vi "4461 - Lockin Engine.vi"(8 "error in (no error)":errorcluster, 9 "Reference In":waveform(dbl)[](array[waveform]), 10 "Signal in":waveform(dbl)[](array[waveform]), 11 "Lockin":refnum<class "Instrument.Lockin.lvclass">) -> (0 "error out":errorcluster, 1 "filter fC (Hz)":dbl=0.3183098861837907, 2 "Results (X,Y,R,Theta)":dbl[][](array[numeric]), 3 "Lockin out":refnum<class "Instrument.Lockin.lvclass">)   [LabVIEW 2016, in "LockinDAQ.lvclass"]
uses:
  LockinDAQ.lvclass
  <vilib>/Analysis/NI_AALBase.lvlib
  <vilib>/Analysis/baseanly.llb/Mean (DBL).vi
  Instrument.Lockin/Instrument.Lockin.lvclass
  C:/Program Files (x86)/National Instruments/LabVIEW 2016/user.lib/LevyLab/Levylab Instruments/SMOs/Instrument/Instrument.lvclass
  C:/Program Files (x86)/National Instruments/LabVIEW 2016/user.lib/LevyLab/Levylab Instruments/SMOs/LevyLab/LevyLab.lvclass
  C:/Program Files (x86)/National Instruments/LabVIEW 2016/vi.lib/JKI/JKI SMO/SMO/SMO.lvclass
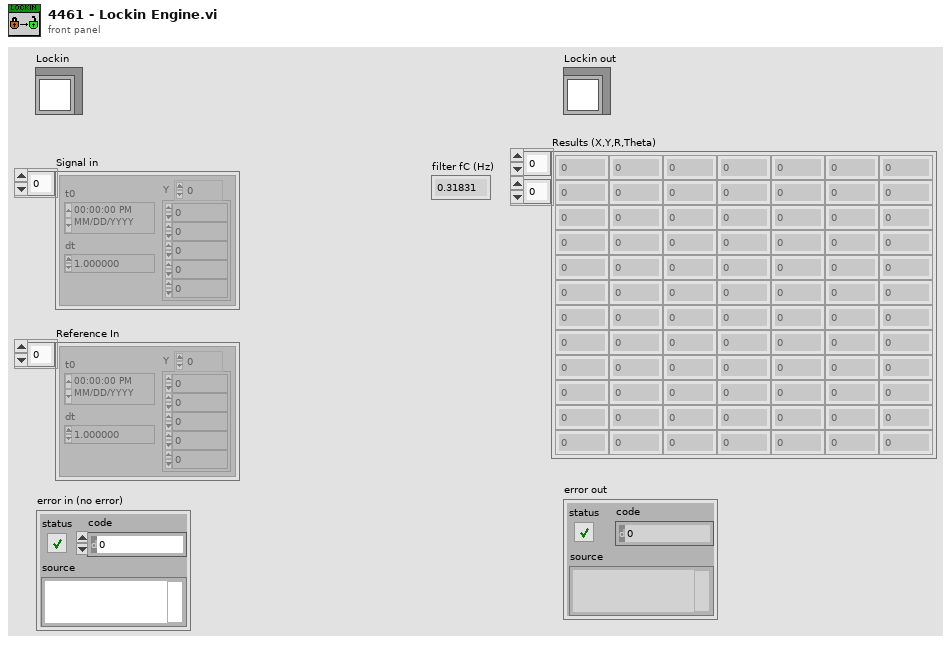
[diagram p1: front panel]
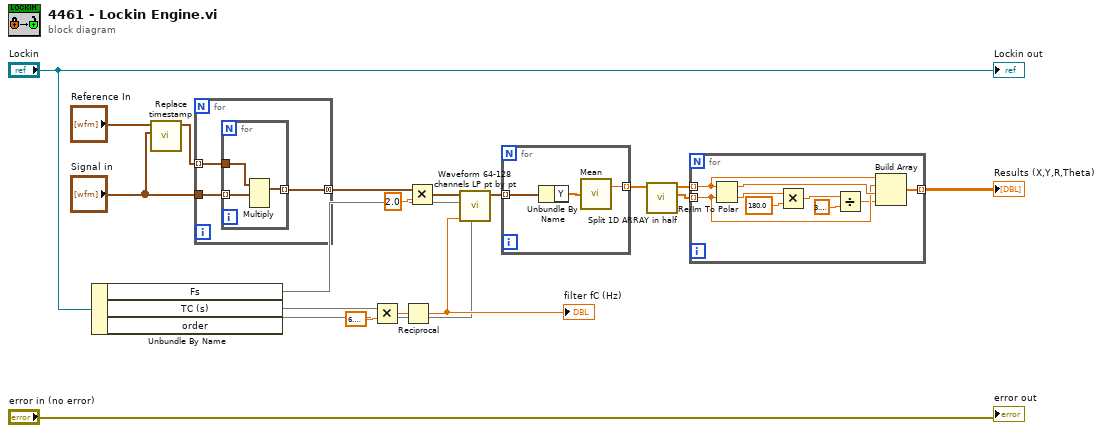
[diagram p0: block diagram]
diagram:
  n1 = Unbundle By Name("Lockin") -> ("Fs"=w6, "TC (s)"=w5, "order"=w2)
  n2 = call "Replace timestamp.vi"("Array in"="Signal in", "Array 2"="Reference In") -> ("Array"=w12:waveform(dbl)[])  [unwired: 9 in]
  n3 = for {
    tunnel: [w22] -> w7 mode=concatenating
    tunnel: w12 -> [w21] mode=indexing
    tunnel: "Signal in" -> [w20]
    n4 = for {
      tunnel: w20 -> [w24] mode=indexing
      tunnel: w21 -> [w23]
      tunnel: [w25] -> w22 mode=indexing
      n5 = Multiply(1:w24, 2:w23) -> (0:w25:waveform(dbl))  [unwired: 1 in, 1 out]
    }
  }
  n6 = Multiply(x=w5, y=6.283185307179586) -> (x*y=w11:dbl)
  n7 = Reciprocal(x=w11) -> (1/x=w13:dbl)
  "filter fC (Hz)" <- w13
  n8 = Multiply(x=w7, y=2.0) -> (x*y=w19:waveform(dbl)[])
  n9 = call "Waveform 64-128 channels LP pt by pt.vi"("order"=w2, "fl"=w13, "fs"=w6, "Array in"=w19) -> ("Array out"=w14:waveform(dbl)[])  [unwired: 7 in]
  n10 = for {
    tunnel: [w27] -> w15 mode=indexing
    tunnel: w14 -> [w26] mode=indexing
    n11 = Unbundle By Name(w26) -> ("Y"=w28:dbl[])
    n12 = call-poly <vilib>:"Mean.vi"("X"=w28) -> ("mean"=w27:dbl)  [unwired: 1 out]
  }
  n13 = call "Split 1D ARRAY in half.vi"("Array in"=w15) -> ("Array out"=w9:dbl[], "Array 3"=w8:dbl[])  [unwired: 9 in]
  n14 = for {
    tunnel: w8 -> [w34] mode=indexing
    tunnel: w9 -> [w36] mode=indexing
    tunnel: [w35] -> w1 mode=indexing
    n15 = Re/Im To Polar(2:w36, 3:w34) -> (0:w32:dbl, 1:w37:dbl)
    n16 = Multiply(x=w32, y=180.0) -> (x*y=w33:dbl)
    n17 = Divide(x=w33, y=3.141592653589793) -> (x/y=w29:dbl)
    n18 = Build Array(w34, w36, w37, w29) -> (w35:dbl[])
  }
  "Results (X,Y,R,Theta)" <- w1
  "Lockin out" <- "Lockin"
  "error out" <- "error in (no error)"
